vi "Generate from Log Data.vi"(0 "TDMS controls in":T1[][](array[typedef]), 1 "Samples per Write":u32=1024000 format="%.3p", 5 "HSS Resource references":refnum<k20>[](array[refnum]), 9 "Queue in":refnum<queue>, 11 "error in":errorcluster, 12 "Infinite Gene":bool, 13 "Previewed Channel":T2) -> (3 "Channels Running?":bool[](array[boolean]), 4 "TDMS controls out":T1[][](array[typedef]), 6 "Enough Space":bool, 8 "Asynchronous \nRead Finished?":bool, 10 "Queue out":refnum<queue>, 15 "error out":errorcluster)   [LabVIEW 2018]
uses:
  TypeDefs/TDMS read.ctl
  TDMS Raw to Channels/Previewed Channel - Enum.ctl
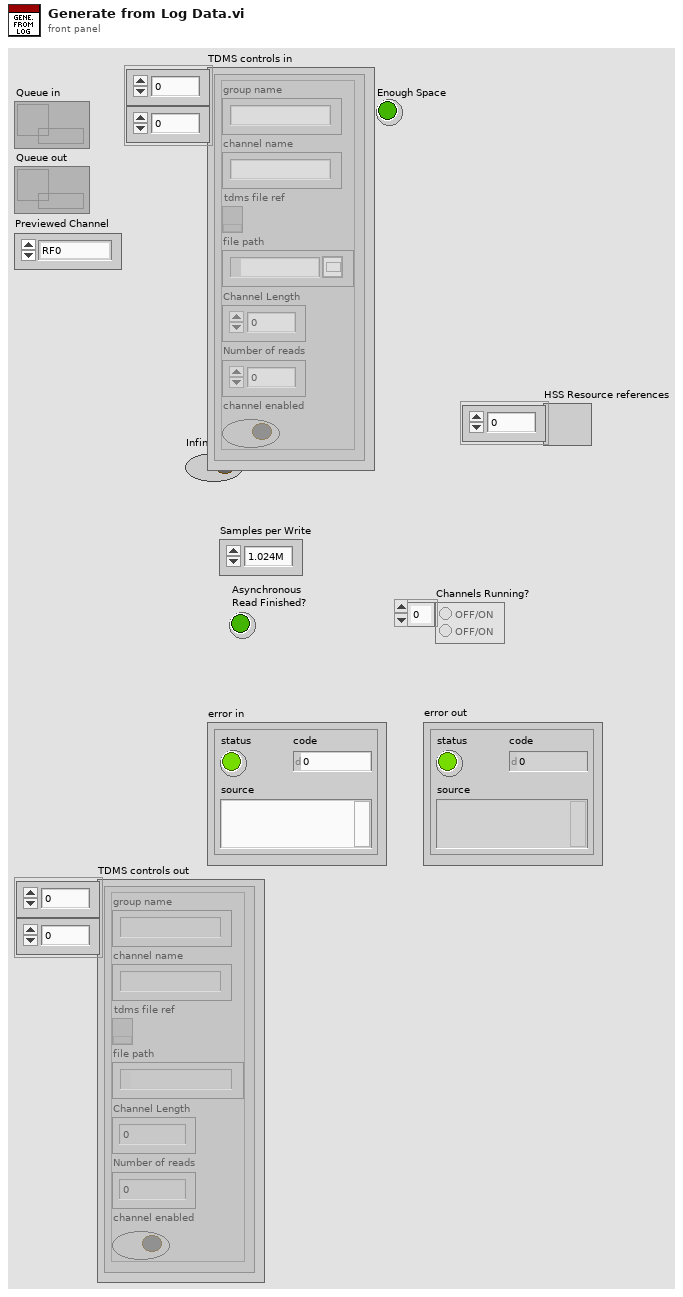
[diagram p1: front panel]
types:
  T1 = typedef "TDMS read.ctl" = cluster{"group name":string, "channel name":string, "tdms file ref":refnum<k34>, "file path":path, "Channel Length":i64, "Number of reads":i64, "channel enabled":bool}
  T2 = typedef "Previewed Channel - Enum.ctl" = enum16{"RF0", "RF1"}
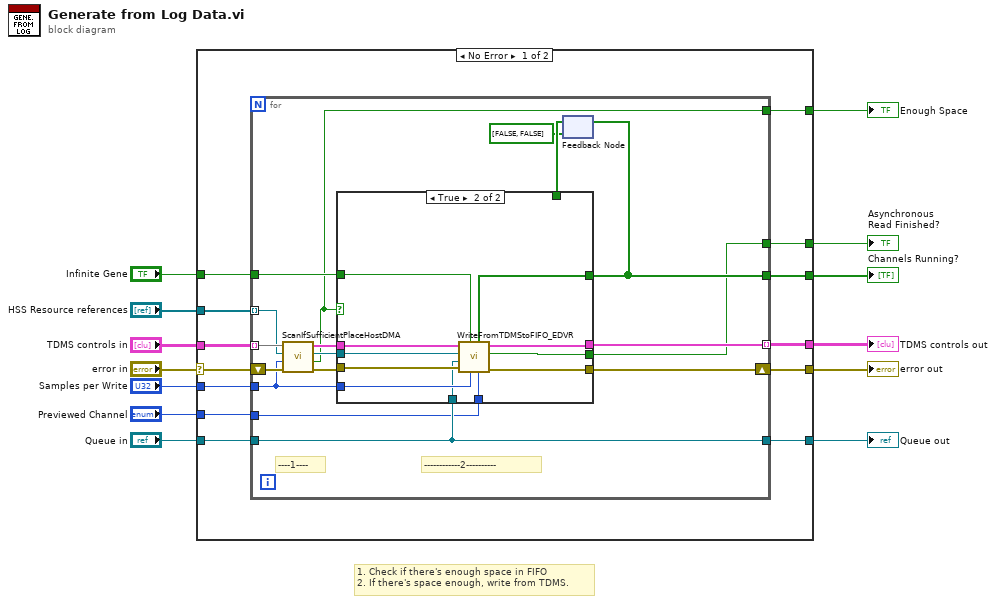
[diagram p0: block diagram]
diagram:
  # "1. Check if there's enough space in FIFO\n2. If there's space enough, write from TDMS."
  n1 = case shown="No Error" "error in" {
    selector: "error in" -> [w25 w60]
    tunnel: [w26 w60] -> w13
    tunnel: "Samples per Write" -> [w24 _]
    tunnel: [w23 _] -> w10
    tunnel: [w22 _] -> w9
    tunnel: "Infinite Gene" -> [w21 _]
    tunnel: "HSS Resource references" -> [w20 _]
    tunnel: "TDMS controls in" -> [w19 w58]
    tunnel: "Queue in" -> [w18 w59]
    tunnel: [w17 w59] -> w4
    tunnel: "Previewed Channel" -> [w16 _]
    tunnel: [w15 _] -> w2
    tunnel: [w14 w58] -> w1
    frame No Error {
      n2 = for {
        tunnel: w20 -> [w34] mode=indexing
        tunnel: w24 -> [w31]
        tunnel: [w43] -> w23
        tunnel: [w27] -> w22
        tunnel: w21 -> [w40]
        shift-right: [w33] -> w26
        shift-left: w25 -> [w38]
        tunnel: w19 -> [w39] mode=indexing
        tunnel: w18 -> [w32]
        tunnel: [w32] -> w17
        tunnel: w16 -> [w30]
        tunnel: [w29] -> w15
        tunnel: [w28] -> w14 mode=indexing
        # "------------2----------"
        # "----1----"
        n3 = call "ScanIfSufficientPlaceHostDMA.vi"("error in (no error)"=w38, "Samples per Write"=w31, "HSS Resource reference"=w34, "TDMS controls in"=w39) -> ("error out"=w36:errorcluster, "Enough Space"=w29:bool, "HSS Resource reference out"=w35:refnum<k20>, "TDMS controls out"=w37:T1[])  [unwired: 4 in]
        n4 = feedback #1(bool[] [FALSE, FALSE] ("Channels Running?")) -> (w42:bool[])
        n5 = case shown="True" w29 {
          tunnel: [w46 w57] -> w33
          tunnel: w37 -> [w44 w53]
          tunnel: w35 -> [_ w52]
          tunnel: w36 -> [w46 w56]
          tunnel: w31 -> [_ w50]
          tunnel: [w45 w55] -> w43
          tunnel: w42 -> [w45 _]
          tunnel: w40 -> [_ w54]
          tunnel: [_ w51] -> w27
          tunnel: w32 -> [_ w49]
          tunnel: w30 -> [_ w48]
          tunnel: [w44 w47] -> w28
          frame False {
          }
          frame True {
            n6 = call "WriteFromTDMStoFIFO_EDVR.vi"("Previewed Channel"=w48, "Samples per Write"=w50, "Infinite Generation"=w54, "error in (no error)"=w56, "Queue in"=w49, "HSS refnum in"=w52, "TDMS read controls in"=w53) -> ("error out"=w57:errorcluster, "read process finished?"=w51:bool, "TDMS read controls out"=w47:T1[], "Channels Running?"=w55:bool[])  [unwired: 1 in]
          }
        }
        n7 = feedback-in #1(w43) -> ()
      }
    }
    frame Error {
    }
  }
  "error out" <- w13
  "Channels Running?" <- w10
  "Asynchronous \nRead Finished?" <- w9
  "Queue out" <- w4
  "Enough Space" <- w2
  "TDMS controls out" <- w1
